vi "CU_testCommittee.vi"(0 "ClassifierClass in":refnum<class "ClassifierClass.lvclass">, 1 "Classifier Refs in":T2[](array[typedef]), 2 "Indices":i8[](array[numeric]), 3 "error in":errorcluster, 4 "Classification Distribution":i32[][][](array[numeric]), 5 "DataTypes":T1=enum."Test Data") -> (6 "ClassifierClass out":refnum<class "ClassifierClass.lvclass">, 7 "Confusion Matrix":i32[][](array[numeric]), 8 "Accuracy":dbl, 9 "error out":errorcluster)   [LabVIEW 2016, in "Classifier.lvlib" / "ClassifierClass.lvclass"]
uses:
  ClassifierClass.lvclass
  <vilib>/vision/Classification.llb/IMAQ Classifier Session.ctl
  CU_DataTypes.ctl
  ClassifierClass.lvclass/ClassifierClass.ctl
  CU_CohenKappa.vi
  <vilib>/vision/NI_Vision_Development_Module.lvlib
  <vilib>/addons/Machine Learning/NILabs_MLT.lvlib
  Classifier.lvlib
panel:
  # "This VI is a part of BCI Design library, http://www.ru-bci.org \nCopyright © 2020, Sotnikov Peter, All rights reserved. License: CC BY-NC 4.0"
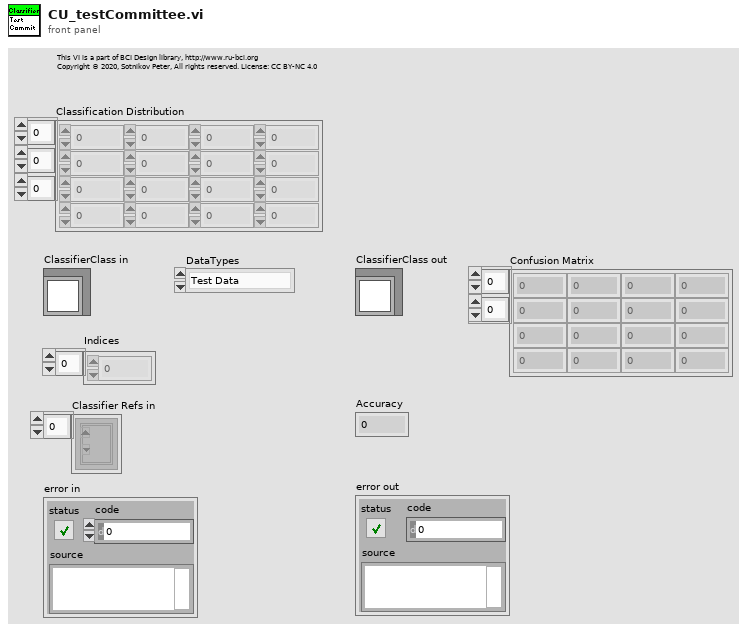
[diagram p1: front panel]
types:
  T1 = typedef "Classifier.lvlib/CU_DataTypes.ctl" = enum16{"Training Data", "Test Data", "Training Data (cross-check)", "Test Data (cross-check)"}
  T2 = typedef "IMAQ Classifier Session.ctl" = refnum<k1>
  T3 = typedef "Classifier.lvlib/CU_ClassifierQualityMeasure.ctl" = enum16{"Accuracy", "Cohen's kappa"}
  T4 = typedef "XML_EEG_Features.lvlib/XML_FF_Trial.ctl" = cluster{"ClassLabel":string, "FeatureVector":dbl[]}
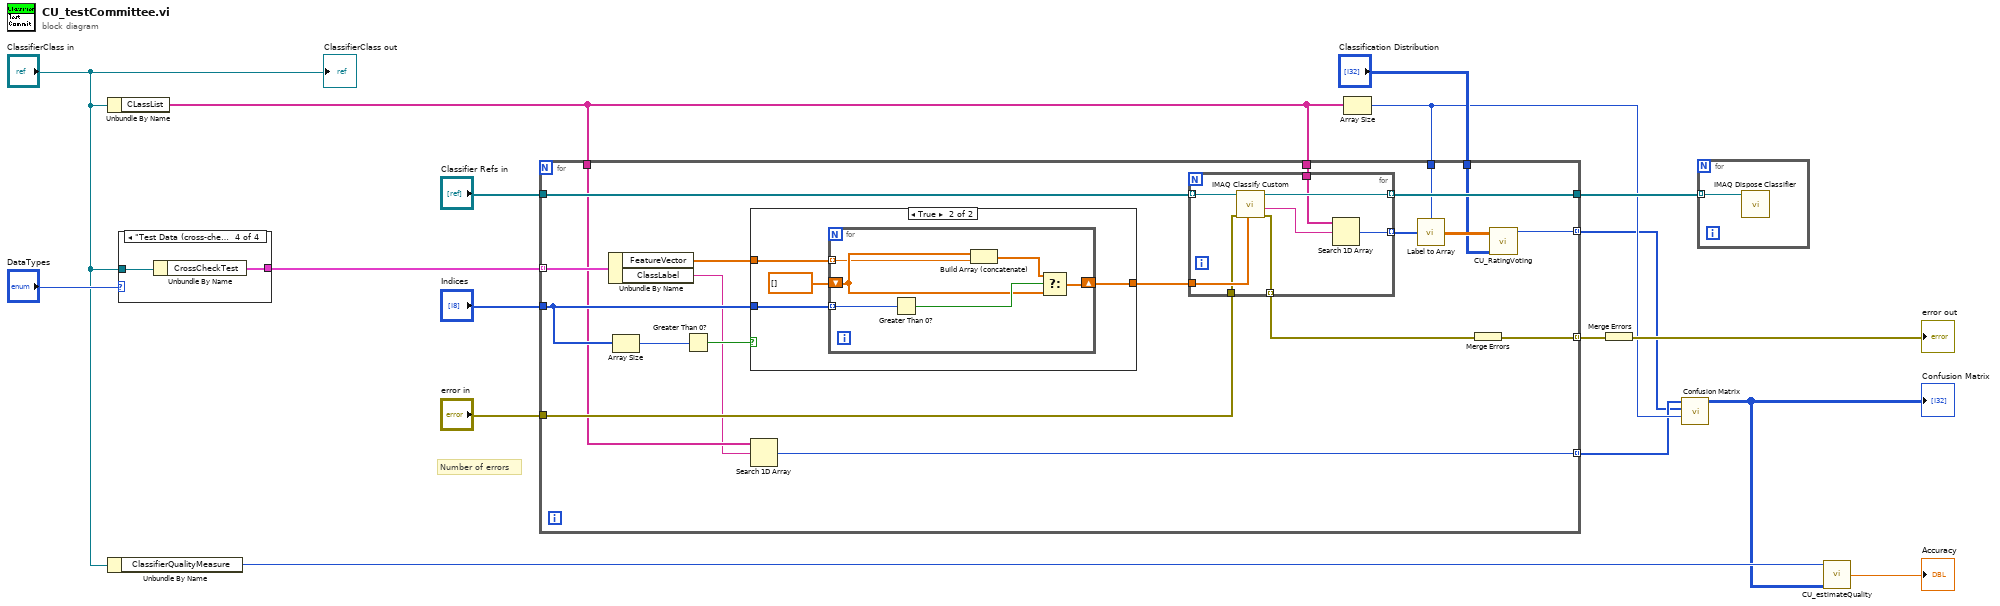
[diagram p0: block diagram]
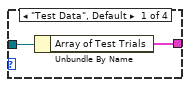
[diagram p2: hidden frame]
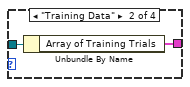
[diagram p3: hidden frame]
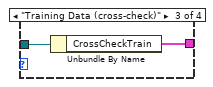
[diagram p4: hidden frame]
diagram:
  # "Number of errors"
  n1 = Unbundle By Name("ClassifierClass in") -> ("CLassList"=w11:string[])
  n2 = Unbundle By Name("ClassifierClass in") -> ("ClassifierQualityMeasure"=w3:T3)
  n3 = case shown="\"Test Data (cross-check)\"" "DataTypes" {
    tunnel: "ClassifierClass in" -> [w19 w21 w23 w25]
    tunnel: [w18 w20 w22 w24] -> w7
    frame "Test Data", Default {
      n4 = Unbundle By Name(w19) -> ("Array of Test Trials"=w18:T4[])
    }
    frame "Training Data" {
      n5 = Unbundle By Name(w21) -> ("Array of Training Trials"=w20:T4[])
    }
    frame "Training Data (cross-check)" {
      n6 = Unbundle By Name(w23) -> ("CrossCheckTrain"=w22:T4[])
    }
    frame "Test Data (cross-check)" {
      n7 = Unbundle By Name(w25) -> ("CrossCheckTest"=w24:T4[])
    }
  }
  n8 = Array Size(array=w11) -> (size(s)=w9:i32)
  n9 = for {
    tunnel: "Classifier Refs in" -> [w40]
    tunnel: w7 -> [w43] mode=indexing
    tunnel: "Indices" -> [w41]
    tunnel: "error in" -> [w38]
    tunnel: [w35] -> w14 mode=indexing
    tunnel: [w37] -> w12
    tunnel: w11 -> [w34]
    tunnel: w11 -> [w33]
    tunnel: w9 -> [w30]
    tunnel: "Classification Distribution" -> [w28]
    tunnel: [w27] -> w4 mode=indexing
    tunnel: [w26] -> w5 mode=indexing
    n10 = Unbundle By Name(w43) -> ("FeatureVector"=w42:dbl[], "ClassLabel"=w32:string)
    n11 = Array Size(array=w41) -> (size(s)=w45:i32)
    n12 = Greater Than 0?(x=w45) -> (x > 0?=w44:bool)
    n13 = case shown="True" w44 {
      tunnel: w42 -> [w54 w58]
      tunnel: w41 -> [_ w57]
      tunnel: [w54 w55] -> w39
      frame False {
      }
      frame True {
        n14 = for {
          tunnel: w58 -> [w60] mode=indexing
          tunnel: w57 -> [w64] mode=indexing
          shift-right: [w63] -> w55
          shift-left: dbl[] [] -> [w61]
          n15 = Greater Than 0?(x=w64) -> (x > 0?=w62:bool)
          n16 = Build Array (concatenate)(w61, w60) -> (w59:dbl[])
          n17 = Select(t=w59, s=w62, f=w61) -> (s? t:f=w63:dbl[])
        }
      }
    }
    n18 = Search 1D Array(1D array=w33, element=w32) -> (index of element=w26:i32)  [unwired: 1 in]
    n19 = for {
      tunnel: w40 -> [w53] mode=indexing
      tunnel: w39 -> [w52]
      tunnel: w38 -> [w51]
      tunnel: [w50] -> w36 mode=indexing
      tunnel: [w49] -> w37 mode=indexing
      tunnel: w34 -> [w48]
      tunnel: [w46] -> w31 mode=indexing
      n20 = call "IMAQ Classify Custom"("Feature Vector"=w52, "error in (no error)"=w51, "Classifier Session"=w53) -> ("error out"=w50:errorcluster, "Class"=w47:string, "Classifier Session (dup)"=w49:T2)  [unwired: 3 in, 3 out]
      n21 = Search 1D Array(1D array=w48, element=w47) -> (index of element=w46:i32)  [unwired: 1 in]
    }
    n22 = call <vilib>:"Label to Array.vi"("Classes"=w31, "# of classes"=w30) -> ("Array"=w29:dbl[][])
    n23 = Merge Errors(w36) -> (w35:errorcluster)
    n24 = call "CU_RatingVoting.vi"("Classification Distribution"=w28, "IndicatorMatrix"=w29) -> ("Class Index"=w27:i32)  [unwired: 9 in]
  }
  n25 = Merge Errors(w14) -> (→"error out":errorcluster)
  n26 = call <vilib>:"Confusion Matrix.vi"("# of classes"=w9, "Predicted class labels"=w4, "Actual class labels"=w5) -> ("Confusion Matrix"=w2:i32[][])  [unwired: 7 in, 1 out]
  "Confusion Matrix" <- w2
  n27 = for {
    tunnel: w12 -> [w65] mode=indexing
    n28 = call "IMAQ Dispose Classifier"("Classifier Session"=w65) -> ()  [unwired: 10 in, 1 out]
  }
  n29 = call "CU_estimateQuality.vi"("Quality Measure in"=w3, "Confusion Matrix in"=w2) -> ("Classification Quality out"=→"Accuracy":dbl)  [unwired: 6 in]
  "ClassifierClass out" <- "ClassifierClass in"
